vi "SQL_CreateUser.vi"(9 "UsersTable":string, 11 "ConnectionDSN":string) -> ()   [LabVIEW 2017]
panel:
  in  "Cancel Button":bool
  in  "OK Button":bool
  in  "Role":u16(ring) items=["Operator", "Team Leader", "Technician", "Supervisor", "Engineer", "Assistant Manager", "Manager", "Director", "C-Suite"]
  in  "Departments":u16(ring) items=["Maintenance", "Process Engineering", "Production", "Quality"]
  in  "Level":u16(ring) items=["0", "1", "2", "3", "4", "5"]
  in  "Password":string
  in  "UserName":string
  # "Por favor, escriba sus datos para el registro"
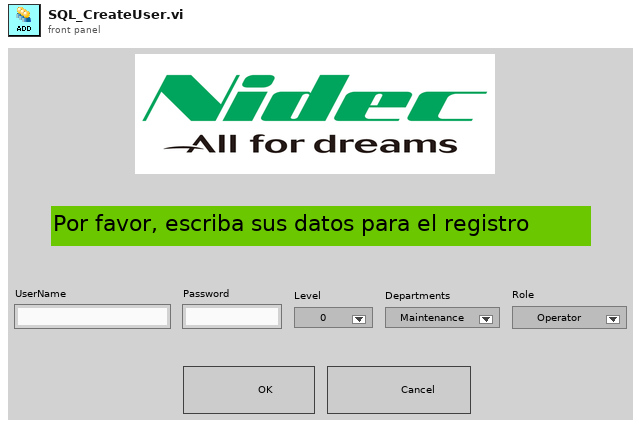
[diagram p1: front panel]
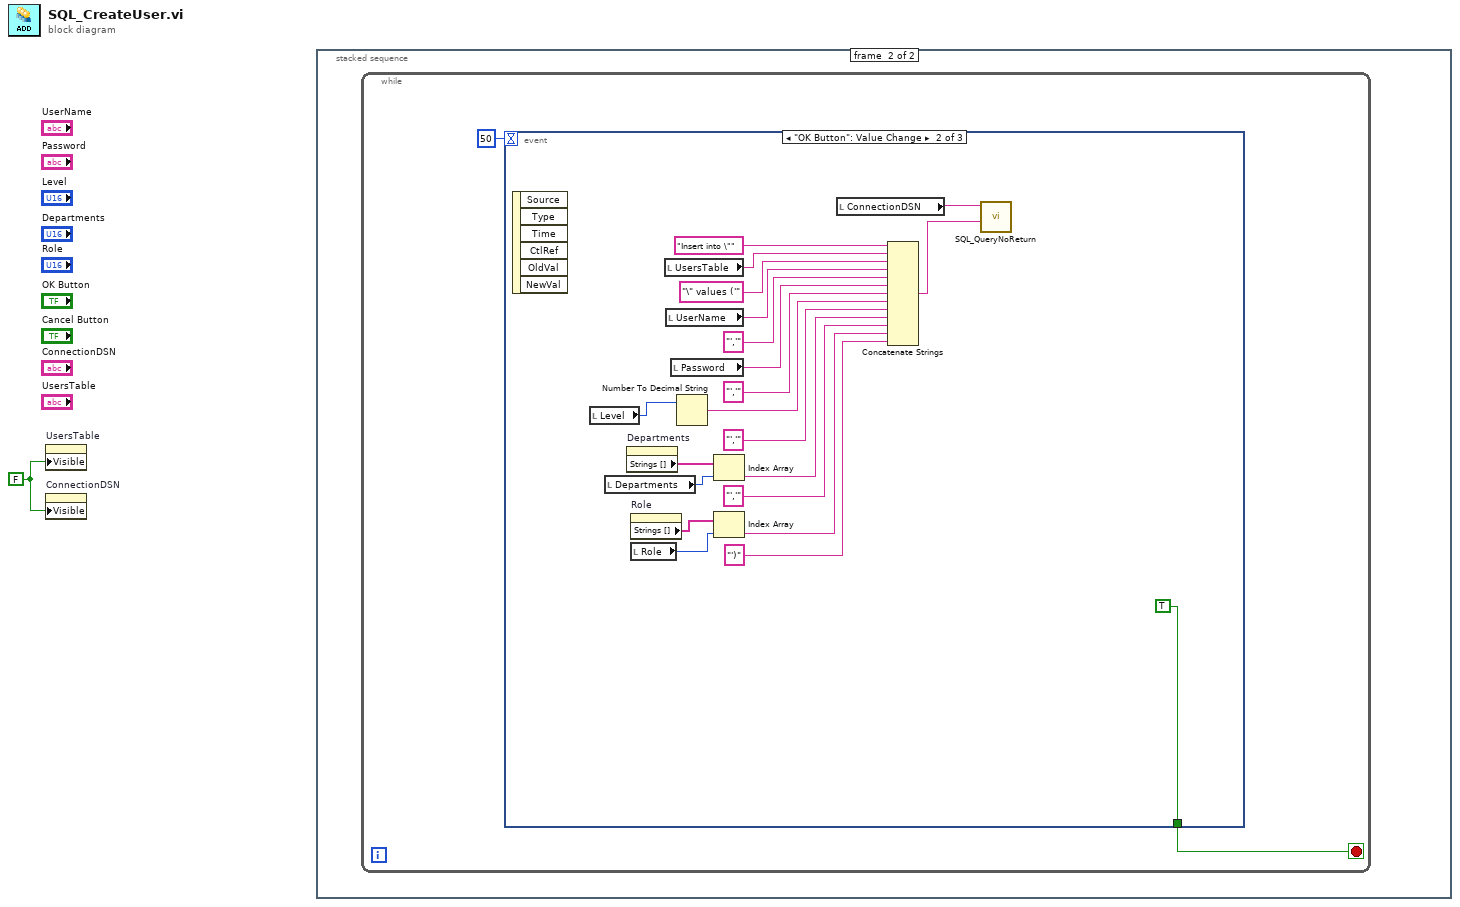
[diagram p0: block diagram]
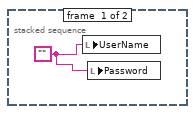
[diagram p2: hidden frame]
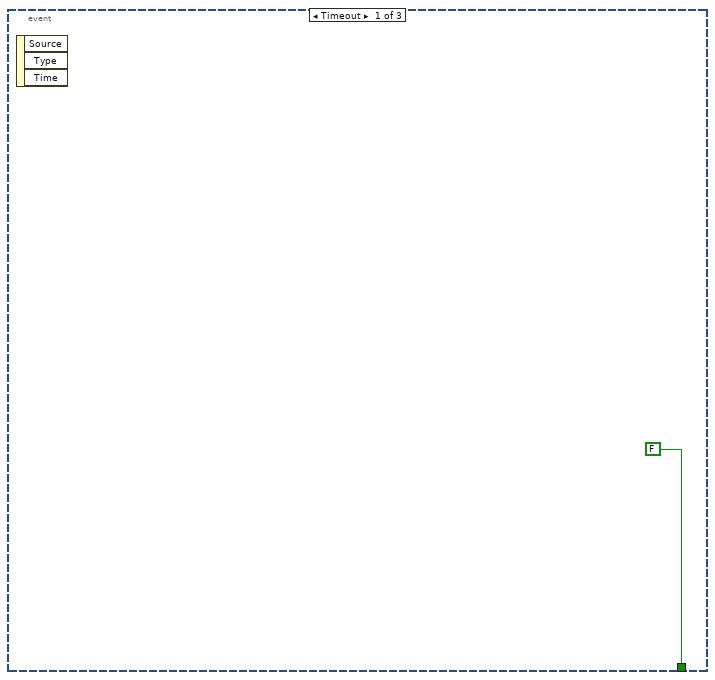
[diagram p3: hidden frame]
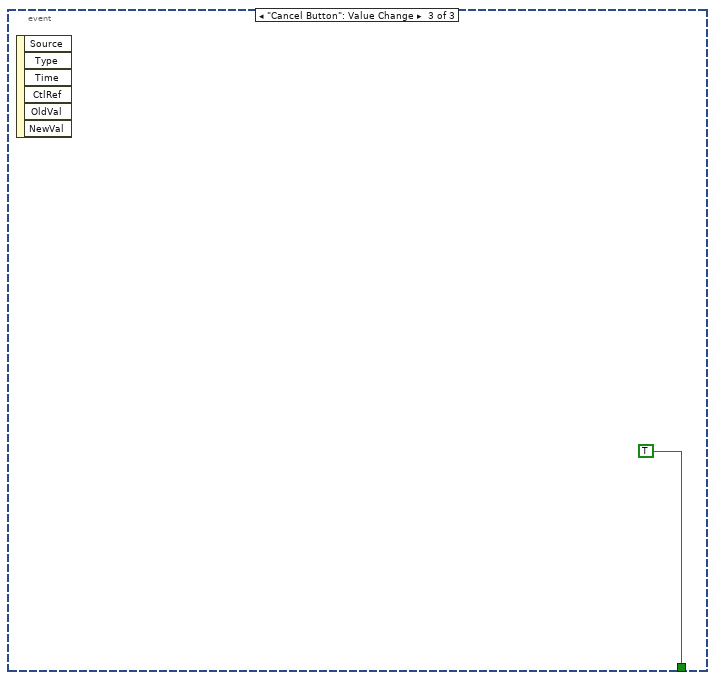
[diagram p4: hidden frame]
diagram:
  w1 = FALSE
  n1 = property on="UsersTable" class="Str"("Visible"=w1) -> ()  [unwired: 2 in, 2 out]
  n2 = property on="ConnectionDSN" class="Str"("Visible"=w1) -> ()  [unwired: 2 in, 2 out]
  n3 = stacked-sequence {
    frame #0 {
      w2 = ""
      n4 = local write "UserName"(w2) -> ()
      n5 = local write "Password"(w2) -> ()
    }
    frame #1 {
      n6 = while {
        stop <- w3 stop-if-true
        n7 = event shown="[1] \"OK Button\": Value Change" {
          selector: _ -> [_ _ _]
          dyn-events: _ -> [_ _ _]
          timeout: 50 -> [_ _ _]
          tunnel: [FALSE TRUE TRUE] -> w3
          event Timeout {
            n8 = event-data() -> ()  [unwired: 1 in, 3 out]
          }
          event "OK Button": Value Change {
            n9 = event-data() -> ()  [unwired: 1 in, 6 out]
            n10 = local read "Level"() -> (w13:u16)
            n11 = local read "Departments"() -> (w23:u16)
            n12 = property on="Departments" class="Ring (strict)"() -> ("Strings []"=w24:string[])  [unwired: 2 in, 2 out]
            n13 = property on="Role" class="Ring (strict)"() -> ("Strings []"=w22:string[])  [unwired: 2 in, 2 out]
            n14 = local read "Role"() -> (w21:u16)
            n15 = local read "UsersTable"() -> (w19:string)
            n16 = local read "UserName"() -> (w17:string)
            n17 = local read "Password"() -> (w15:string)
            n18 = Number To Decimal String(number=w13) -> (decimal integer string=w12:string)  [unwired: 1 in]
            n19 = Index Array(array=w24, index=w23) -> (element=w10:string)
            n20 = Index Array(array=w22, index=w21) -> (element=w8:string)
            n21 = local read "ConnectionDSN"() -> (w25:string)
            n22 = Concatenate Strings("Insert into \"", w19, "\" values ('", w17, "','", w15, "','", w12, "','", w10, "','", w8, "')") -> (w6:string)
            n23 = call "SQL_QueryNoReturn.vi"("SQL query"=w6, "ConnectionDSN"=w25) -> ()  [unwired: 10 in]
          }
          event "Cancel Button": Value Change {
            n24 = event-data() -> ()  [unwired: 1 in, 6 out]
          }
        }
      }
    }
  }
